vi "dfd_Build Floating Filter from Coef.vi"(6 "fs [Hz]":dbl=1.0, 8 "error in (no error)":errorcluster, 10 "filter coef":T2, 11 "filter in":T1={"mSRate_Fs"=1.0, "mSRate_Version"="1.0", "mSRate_Comments"="", "mSRate_OrgCoef"={"type"=enum."Undefined", "gain"=1.0, "coef a (k)"=[], "coef b (v)"=[]}, "mSRate_CurCoef"={"type"=enum."Undefined", "gain"=1.0, "coef a (k)"=[], "coef b (v)"=[]}, "mSRate_Quantized?"=FALSE, "mSRate_QCoef"={"type"=enum."Undefined", "gain"=1.0, "coef a (k)"=[], "coef b (v)"=[]}, "mSRate_QSettings"=[], "mSRate_Order"=0, "mSRate_Scaling"={"mSRate_ScaleByPowerOf2?"=FALSE, "mSRate_ScaleType"=enum."No Norm"}} {"mSRate_QSettings"."source" items=["Coef a/k"=0, "Coef b/v"=7, "Input"=1, "Output"=2, "Multiplicand"=3, "Product"=4, "Sum"=5, "Delay"=6, "Gain"=8]}) -> (0 "error out":errorcluster, 3 "filter out":T1={"mSRate_Fs"=1.0, "mSRate_Version"="1.0", "mSRate_Comments"="", "mSRate_OrgCoef"={"type"=enum."Undefined", "gain"=1.0, "coef a (k)"=[], "coef b (v)"=[]}, "mSRate_CurCoef"={"type"=enum."Undefined", "gain"=1.0, "coef a (k)"=[], "coef b (v)"=[]}, "mSRate_Quantized?"=FALSE, "mSRate_QCoef"={"type"=enum."Undefined", "gain"=1.0, "coef a (k)"=[], "coef b (v)"=[]}, "mSRate_QSettings"=[], "mSRate_Order"=0, "mSRate_Scaling"={"mSRate_ScaleByPowerOf2?"=FALSE, "mSRate_ScaleType"=enum."No Norm"}} {"mSRate_QSettings"."source" items=["Coef a/k"=0, "Coef b/v"=7, "Input"=1, "Output"=2, "Multiplicand"=3, "Product"=4, "Sum"=5, "Delay"=6, "Gain"=8]})   [LabVIEW 2017, in "NI_DigFilterLicensed.lvlib"]
uses:
  <vilib>/addons/Digital Filter Design/NI_DigFilterLicensed.lvlib
  <vilib>/addons/Digital Filter Design/_Objects.llb/DFD Filter Obj.ctl
  <vilib>/addons/Digital Filter Design/_Objects.llb/DFD Filter Coef.ctl
  <vilib>/addons/Digital Filter Design/_Objects.llb/DFD Filter Structure Type Selector.ctl
  <vilib>/addons/Digital Filter Design/_Objects.llb/dfd_Internal Quantization Settings.ctl
  <vilib>/addons/Digital Filter Design/_Objects.llb/dfd_Internal Quantization Srcs.ctl
  <vilib>/addons/Digital Filter Design/_Objects.llb/DFD Coef Norm Type.ctl
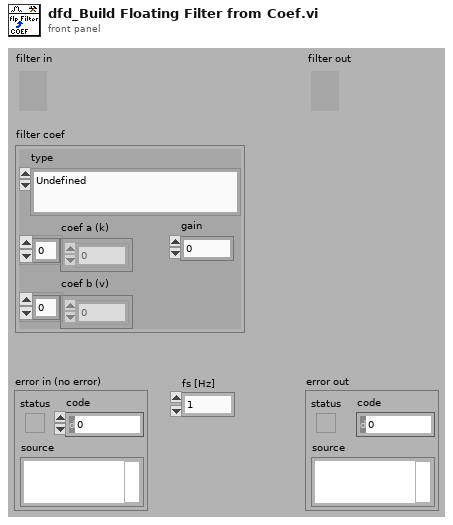
[diagram p1: front panel]
types:
  T1 = typedef "NI_DigFilterLicensed.lvlib/DFD Filter Obj.ctl" = cluster{"mSRate_Fs":dbl, "mSRate_Version":string, "mSRate_Comments":string, "mSRate_OrgCoef":T2, "mSRate_CurCoef":T2, "mSRate_Quantized?":bool, "mSRate_QCoef":T2, "mSRate_QSettings":T4[], "mSRate_Order":i32, "mSRate_Scaling":cluster{"mSRate_ScaleByPowerOf2?":bool, "mSRate_ScaleType":T6}}
  T2 = typedef "NI_DigFilterLicensed.lvlib/DFD Filter Coef.ctl" = cluster{"type":T3, "gain":dbl, "coef a (k)":dbl[], "coef b (v)":dbl[]}
  T3 = typedef "NI_DigFilterLicensed.lvlib/DFD Filter Structure Type Selector.ctl" = enum16{"Undefined", "FIR Direct Form", "FIR Direct Form Transposed", "FIR Symmetric", "FIR Antisymmetric", "IIR Direct Form I", "IIR Direct Form I Transposed", "IIR Direct Form II", "IIR Direct Form II Transposed", "IIR Cascaded Second Order Sections Form I", "IIR Cascaded Second Order Sections Form I Transposed", "IIR Cascaded Second Order Sections Form II", "IIR Cascaded Second Order Sections Form II Transposed", "Lattice Allpass (basic sections)", "Lattice Allpass (one multiplier sections)", "Lattice Allpass (normalized sections)", "Lattice AR (basic sections)", "Lattice AR (one multiplier sections)", "Lattice AR (normalized sections)", "Lattice MA (minimum phase)", "Lattice MA (maximum phase)", "Lattice ARMA (basic sections)", "Lattice ARMA (one multiplier sections)", "Lattice ARMA (normalized sections)"}
  T4 = typedef "NI_DigFilterLicensed.lvlib/dfd_Internal Quantization Settings.ctl" = cluster{"source":T5, "wl":i16, "iwl":i16, "overflow mode":enum16{"Saturation", "Wrap"}, "rounding mode":enum16{"Nearest", "Truncation"}, "signed?":bool}
  T5 = typedef "NI_DigFilterLicensed.lvlib/dfd_Internal Quantization Srcs.ctl" = u16
  T6 = typedef "NI_DigFilterLicensed.lvlib/DFD Coef Norm Type.ctl" = enum16{"No Norm", "Time Domain 1-Norm", "Time Domain 2-Norm", "Time Domain Inf-Norm"}
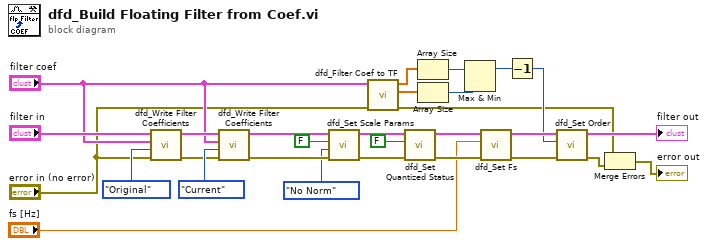
[diagram p0: block diagram]
diagram:
  n1 = call <vilib>:"dfd_Write Filter Coefficients.vi"("error in (no error)"="error in (no error)", "coef source"=enum16{"Original", "Current", "Quantized"}."Original", "filter coef"="filter coef", "filter in"="filter in") -> ("error out"=w24:errorcluster, "filter out"=w23:T1)  [unwired: 6 out]
  n2 = call <vilib>:"dfd_Write Filter Coefficients.vi"("error in (no error)"=w24, "coef source"=enum16{"Original", "Current", "Quantized"}."Current", "filter coef"="filter coef", "filter in"=w23) -> ("error out"=w26:errorcluster, "filter out"=w4:T1)  [unwired: 6 out]
  n3 = call <vilib>:"dfd_Set Scale Params.vi"("scale type"=DFD_Coef_Norm_Type."No Norm", "scale by Power of 2?"=FALSE, "filter in"=w4) -> ("filter out"=w3:T1)  [unwired: 8 out]
  n4 = call <vilib>:"dfd_Filter Coef to TF.vi"("error out"="error in (no error)", "filter coef"="filter coef") -> ("error"=w6:errorcluster, "denominator"=w15:dbl[], "numerator"=w16:dbl[])  [unwired: 7 out]
  n5 = call <vilib>:"dfd_Set Quantized Status.vi"("error in (no error)"=w26, "quantized?"=FALSE, "filter in"=w3) -> ("error out"=w20:errorcluster, "filter out"=w21:T1)  [unwired: 7 out]
  n6 = Array Size(array=w16) -> (size(s)=w14:i32)
  n7 = Array Size(array=w15) -> (size(s)=w13:i32)
  n8 = Max & Min(x=w14, y=w13) -> (max(x,y)=w12:i32)  [unwired: 1 out]
  n9 = call <vilib>:"dfd_Set Fs.vi"("error in (no error)"=w20, "fs [Hz]"="fs [Hz]", "filter in"=w21) -> ("error out"=w10:errorcluster, "filter out"=w11:T1)  [unwired: 7 out]
  n10 = Decrement(x=w12) -> (x-1=w9:i32)
  n11 = call <vilib>:"dfd_Set Order.vi"("error in (no error)"=w10, "order"=w9, "filter in"=w11) -> ("error out"=w7:errorcluster, "filter out"=→"filter out":T1)  [unwired: 7 out]
  n12 = Merge Errors(w6, w7) -> (→"error out":errorcluster)
